vi "CLD 1 Elapsed Time Express Front Panel.vi"() -> ()   [LabVIEW 2019]
doc: "LabVIEW CLD 1 Exercise"
panel:
  in  "error in":errorcluster
  out "error out":errorcluster
  out "Elapsed Time":dbl
  out "Time has Elapsed":bool
  in  "Auto Reset":bool=TRUE
  in  "Reset Button":bool
  in  "Stop VI":bool
  in  "Time Target (s)":dbl=2.0
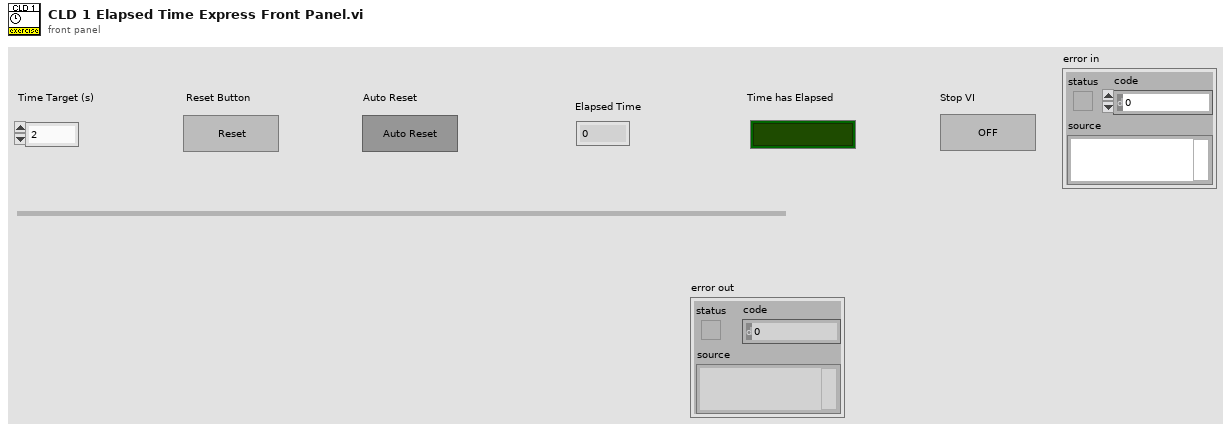
[diagram p1: front panel]
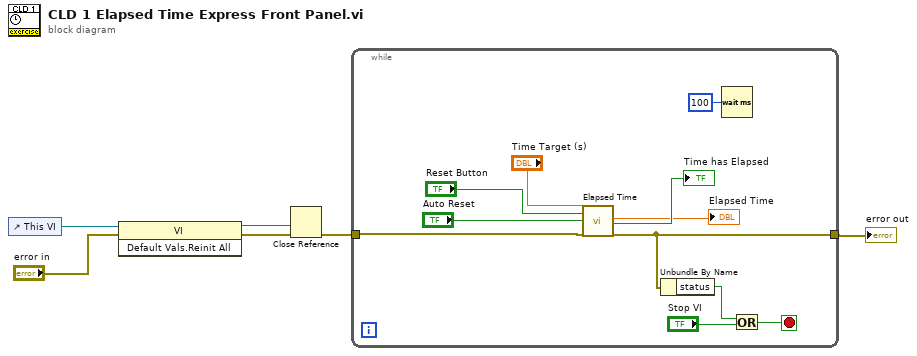
[diagram p0: block diagram]
diagram:
  n1 = control-ref of="This VI"() -> (w5:refnum<vi>)
  n2 = invoke class="VI" method="Default Vals.Reinit All"(reference=w5, error in="error in") -> (reference out=w1:refnum<vi>, error out=w3:errorcluster)  [unwired: 1 in, 1 out]
  n3 = Close Reference(reference=w1, error in (no error)=w3) -> (error out=w2:errorcluster)
  n4 = while {
    tunnel: w2 -> [w13]
    tunnel: [w12] -> w6
    stop <- w9 stop-if-true
    n5 = call "Elapsed Time"("Time Target (s)"="Time Target (s)", "Reset"="Reset Button", "Auto Reset"="Auto Reset", "error in (no error)"=w13) -> ("Elapsed Time (s)"=→"Elapsed Time":dbl, "Time has Elapsed"=→"Time has Elapsed":bool, "error out"=w12:errorcluster)  [unwired: 8 in, 5 out]
    n6 = Unbundle By Name(w12) -> ("status"=w11:bool)
    n7 = Wait (ms)(milliseconds to wait=u32 100) -> ()  [unwired: 1 out]
    n8 = Or(x=w11, y="Stop VI") -> (x .or. y?=w9:bool)
  }
  "error out" <- w6
